vi "VPRebuild.vi"(8 "error in (no error)":errorcluster, 9 "Name of target":string, 10 "Name of build specification":string, 11 "Path to project":path) -> (0 "error out":errorcluster, 2 "Generated files":path[](array[path]))   [LabVIEW 2013, in "VIProject.lvlib"]
uses:
  VIProject.lvlib
  <vilib>/AppBuilder/AB_API_Simple/Build (path).vi
  <vilib>/AppBuilder/AB_API_Simple/NI_App_Builder_API.lvlib
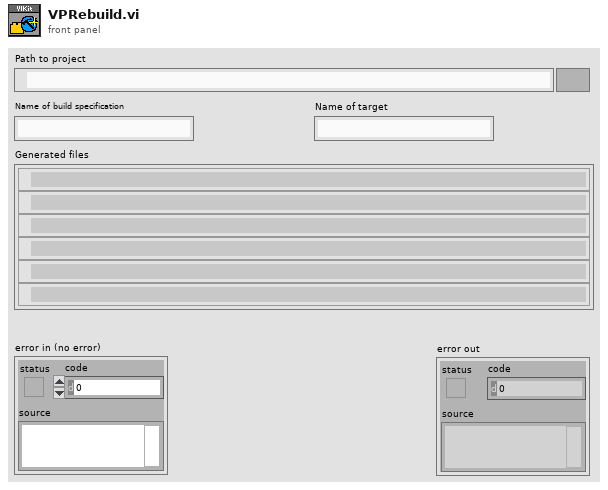
[diagram p1: front panel]
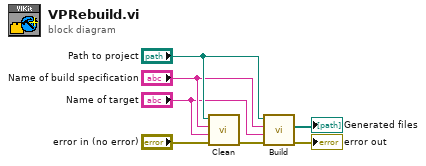
[diagram p0: block diagram]
diagram:
  n1 = call <vilib>:"Clean.vi"("error in (no error)"="error in (no error)", "Name of target (My Computer)"="Name of target", "Name of build specification (if empty: clean all)"="Name of build specification", "Path to project"="Path to project") -> ("error out"=w7:errorcluster)  [unwired: 7 in]
  n2 = call-poly <vilib>:"Build.vi"("error in (no error)"=w7, "Name of target (My Computer)"="Name of target", "Name of build specification (if empty: build all)"="Name of build specification", "Path to project"="Path to project") -> ("error out"=→"error out":errorcluster, "Generated files"=→"Generated files":path[])  [unwired: 6 in]
